vi "Write Record Data.vi"(8 "Error In (no error)":errorcluster, 10 "Record":variant, 11 "Expenses Tracker Saving In":refnum<class "Expenses Tracker Saving.lvclass">) -> (0 "Error Out":errorcluster, 3 "Expenses Tracker Saving Out":refnum<class "Expenses Tracker Saving.lvclass">)   [LabVIEW 2023, in "Expenses Tracker Saving.lvclass"]
uses:
  Expenses Tracker Saving.lvclass
  Ctrls/Saving.ctl
  Expenses Tracker Saving.lvclass/Expenses Tracker Saving.ctl
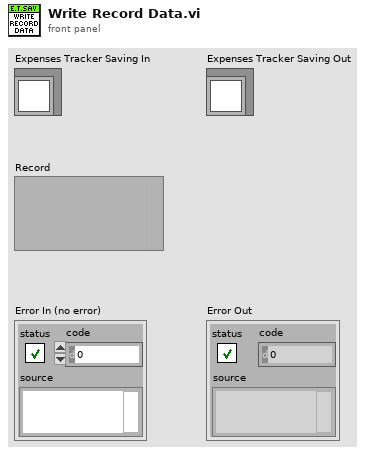
[diagram p1: front panel]
types:
  T1 = typedef "Expenses Tracker Saving.lvclass/Saving.ctl" = cluster{"ID":u32, "Saving_goal":u32, "Value":dbl, "Date_of_entry":timestamp, "Description":string}
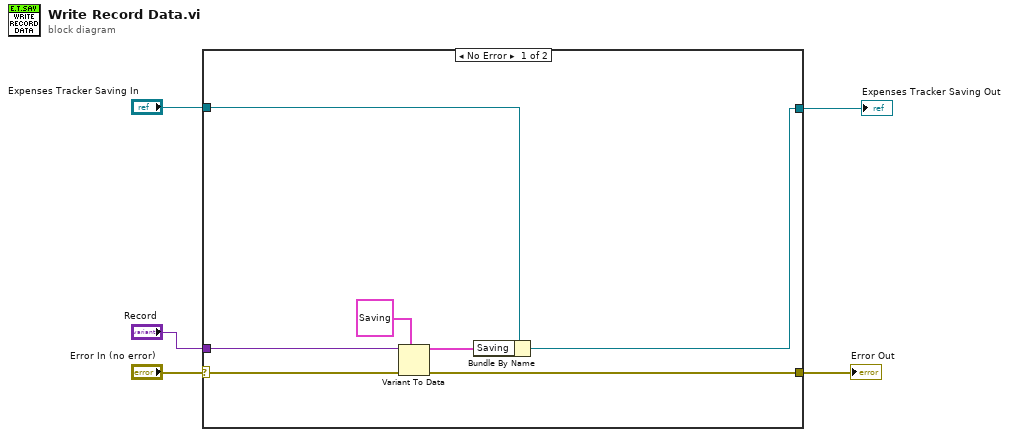
[diagram p0: block diagram]
diagram:
  n1 = case shown="No Error" "Error In (no error)" {
    selector: "Error In (no error)" -> [w10 w14]
    tunnel: [w8 w14] -> w4
    tunnel: [w7 w13] -> w3
    tunnel: "Expenses Tracker Saving In" -> [w6 w13]
    tunnel: "Record" -> [w12 _]
    frame No Error {
      n2 = Variant To Data(error in=w10, type=T1 {"ID"=0, "Saving_goal"=0, "Value"=0.0, "Date_of_entry"=timestamp(0 s since 1904-01-01), "Description"=""} ("Saving"), Variant=w12) -> (data=w11:T1, error out=w8:errorcluster)
      n3 = Bundle By Name(cluster=w6, "Saving"=w11) -> (w7:refnum<class "Expenses Tracker Saving.lvclass">)
    }
    frame Error {
    }
  }
  "Error Out" <- w4
  "Expenses Tracker Saving Out" <- w3
